vi "PlayAndSignalize (SubVI).vi"(8 "Tone (Frequency:Duration)":i32[][](array[numeric]), 9 "State [GYBWR]":bool[](array[boolean]), 10 "Indicators [GYBWR]":refnum<vi>, 11 "LINX Resource":T1) -> ()   [LabVIEW 2014]
uses:
  <vilib>/MakerHub/LINX/Private/Type Defs/LINX Ref.ctl
  <vilib>/MakerHub/LINX/Private/Type Defs/Platform.ctl
  <vilib>/MakerHub/LINX/Private/Type Defs/Interface.ctl
  <vilib>/MakerHub/LINX/Private/Device/Type Defs/LINX Device Config.ctl
  <vilib>/MakerHub/LINX/Private/Device/Type Defs/TCP Config.ctl
  <vilib>/MakerHub/LINX/Private/Device/Type Defs/Channels.ctl
  <vilib>/MakerHub/LINX/LMH-LINX.lvlib
  <vilib>/MakerHub/LINX/Private/Device/Device.lvlib
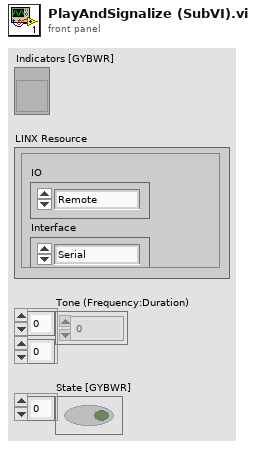
[diagram p1: front panel]
types:
  T1 = typedef "LMH-LINX.lvlib/LINX Ref.ctl" = cluster{"IO":T2, "Interface":T3, "LINX Device Config":T4}
  T2 = typedef "LMH-LINX.lvlib/Platform.ctl" = enum16{"Remote", "Local"}
  T3 = typedef "LMH-LINX.lvlib/Interface.ctl" = enum16{"Serial", "TCP"}
  T4 = typedef "LMH-LINX.lvlib/Device.lvlib/LINX Device Config.ctl" = cluster{"Interface":T3, "COM Port":refnum<visa-resource-name>, "TCP Configuration":T5, "Device Family":u8, "Device ID":u8, "Device Name":string, "TCP Ref":refnum<k5>, "Channels":T6}
  T5 = typedef "LMH-LINX.lvlib/Device.lvlib/TCP Config.ctl" = cluster{"IP Address":string, "Port":u16}
  T6 = typedef "LMH-LINX.lvlib/Channels.ctl" = cluster{"DI":u8[], "DO":u8[], "AI":u8[], "AO":u8[], "PWM":u8[], "QE":u8[], "UART":u8[], "I2C 2":u8[], "SPI":u8[], "CAN":u8[], "Servo":u8[], "AI Ref (V)":dbl, "AI Resolution (Bits)":u8, "AO Ref (V)":dbl, "AO Resolution (Bits)":u8}
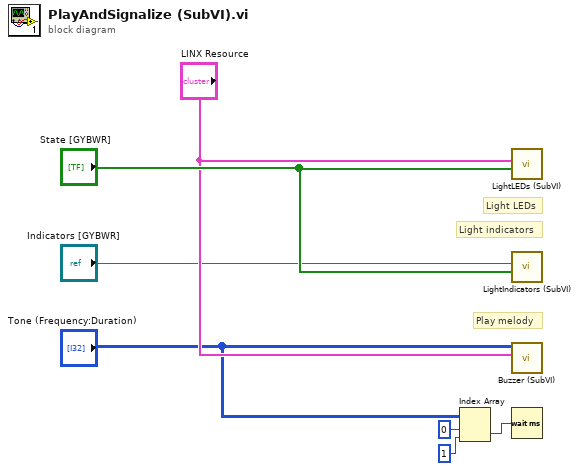
[diagram p0: block diagram]
diagram:
  # "Light LEDs"
  # "Light indicators"
  # "Play melody"
  n1 = Index Array(array="Tone (Frequency:Duration)", index (row)=0, index (col)=1 ("disabled index (col)")) -> (element=w4:i32)
  n2 = call "LightLEDs (SubVI).vi"("Array"="State [GYBWR]", "LINX Resource"="LINX Resource") -> ()  [unwired: 10 in]
  n3 = call "LightIndicators (SubVI).vi"("State [GYBWR]"="State [GYBWR]", "Indicators [GYBWR]"="Indicators [GYBWR]") -> ()  [unwired: 10 in]
  n4 = call "Buzzer (SubVI).vi"("LINX Resource"="LINX Resource", "Melody (frequency:duration)"="Tone (Frequency:Duration)") -> ()  [unwired: 10 in]
  n5 = Wait (ms)(milliseconds to wait=w4) -> ()  [unwired: 1 out]
